vi "current abs pos to rel pos.vi"() -> (2 "rel pos out":cluster{"rel x":dbl, "rel y":dbl, "rel z":dbl}, 3 "abs pos out":cluster{"abs x":dbl, "abs y":dbl, "abs z":dbl})   [LabVIEW 2012]
doc: "SciScan 1.2 160622"
uses:
  <vilib>/Analysis/coordinate.llb/Euler Rotation Order.ctl
  GFG/GFGnumericGet.vi
  GFG/GFGbooleanGet.vi
  <vilib>/Analysis/coordinate.llb/3D Cartesian Coordinate Rotation (Euler) (Scalar).vi
  GFG/GFG library.lvlib
  <vilib>/Analysis/NI_AALPro.lvlib
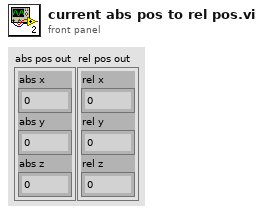
[diagram p1: front panel]
types:
  T1 = cluster{"Xoffset":dbl, "Yoffset":dbl, "Zoffset":dbl}
  T2 = typedef "NI_AALPro.lvlib/Euler Rotation Order.ctl" = u16
  T3 = cluster{"Numeric":dbl, "Numeric":dbl, "Numeric":dbl}
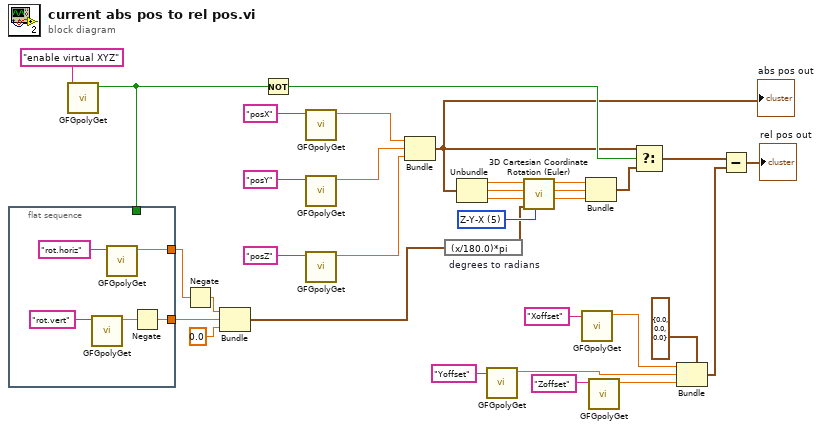
[diagram p0: block diagram]
diagram:
  w26 = T2 5 items=["X-Y-Z", "X-Z-Y", "Y-X-Z", "Y-Z-X", "Z-X-Y", "Z-Y-X", "X-Y-X", "X-Z-X", "Y-X-Y", "Y-Z-Y", "Z-X-Z", "Z-Y-Z"] ("rotation order")
  n1 = flat-sequence {
    tunnel: [w39] -> w29
    tunnel: [w37] -> w27
    tunnel: w13 -> [_]
    frame #0 {
      n2 = call-poly "GFGpolyGet.vi"("Variable Name in"="rot.vert") -> ("Numeric"=w38:dbl)  [unwired: 8 in, 2 out]
      n3 = call-poly "GFGpolyGet.vi"("Variable Name in"="rot.horiz") -> ("Numeric"=w37:dbl)  [unwired: 8 in, 2 out]
      n4 = Negate(x=w38) -> (-x=w39:dbl)
    }
  }
  n5 = call-poly "GFGpolyGet.vi"("Variable Name in"="enable virtual XYZ") -> ("Boolean Value OUT"=w13:bool)  [unwired: 9 in, 1 out]
  n6 = Negate(x=w27) -> (-x=w28:dbl)
  n7 = Bundle(w28, w29, "phi"=0.0) -> (w31:cluster{dbl, dbl, "phi":dbl})  [unwired: 1 in]
  n8 = Not(x=w13) -> (.not. x?=w15:bool)
  n9 = call-poly "GFGpolyGet.vi"("Variable Name in"="posX") -> ("Numeric"=w24:dbl)  [unwired: 8 in, 2 out]
  n10 = call-poly "GFGpolyGet.vi"("Variable Name in"="posY") -> ("Numeric"=w23:dbl)  [unwired: 8 in, 2 out]
  n11 = call-poly "GFGpolyGet.vi"("Variable Name in"="posZ") -> ("Numeric"=w22:dbl)  [unwired: 8 in, 2 out]
  n12 = Bundle("Numeric"=w24, "Numeric"=w23, "Numeric"=w22) -> (w1:T3)  [unwired: 1 in]
  "abs pos out" <- w1
  n13 = expression code="(x/180.0)*pi" "degrees to radians"(w31) -> (w25:cluster{dbl, dbl, "phi":dbl})
  n14 = Unbundle(w1) -> ("Numeric"=w21:dbl, "Numeric"=w20:dbl, "Numeric"=w19:dbl)
  n15 = call-poly "GFGpolyGet.vi"("Variable Name in"="Yoffset") -> ("Numeric"=w7:dbl)  [unwired: 8 in, 2 out]
  n16 = call-poly <vilib>:"3D Cartesian Coordinate Rotation (Euler).vi"("rotation order"=w26, "Euler Angles"=w25, "z"=w19, "y"=w20, "x"=w21) -> ("z out"=w16:dbl, "y out"=w17:dbl, "x out"=w18:dbl)  [unwired: 3 in, 1 out]
  n17 = call-poly "GFGpolyGet.vi"("Variable Name in"="Xoffset") -> ("Numeric"=w8:dbl)  [unwired: 8 in, 2 out]
  n18 = Bundle("x out"=w18, "y out"=w17, "z out"=w16) -> (w14:cluster{"x out":dbl, "y out":dbl, "z out":dbl})  [unwired: 1 in]
  n19 = call-poly "GFGpolyGet.vi"("Variable Name in"="Zoffset") -> ("Numeric"=w6:dbl)  [unwired: 8 in, 2 out]
  n20 = Select(t=w1, s=w15, f=w14) -> (s? t:f=w2:cluster{"x out":dbl, "y out":dbl, "z out":dbl})
  n21 = Bundle(cluster=T1 {"Xoffset"=0.0, "Yoffset"=0.0, "Zoffset"=0.0} ("output cluster"), "Xoffset"=w8, "Yoffset"=w7, "Zoffset"=w6) -> (w4:T1)
  n22 = Subtract(x=w2, y=w4) -> (x-y=→"rel pos out":cluster{dbl, dbl, dbl})
